vi "RP100 CLI Build.vi"(8 "Package Source Folder":path, 9 "Package Version":string="1.5.0.3") -> (0 "error out":errorcluster)   [LabVIEW 2019]
uses:
  <userlib>/LevyLab/Build Support/Build/Typedefs/Build Spec Type--combo.ctl
  <userlib>/LevyLab/Build Support/Build/Build.lvlib
panel:
  in  "error in":errorcluster
  out "project path":string
  out "repository path":string
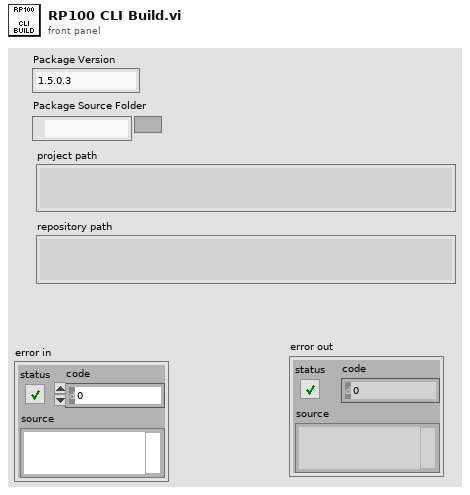
[diagram p1: front panel]
types:
  T1 = typedef "Build.lvlib/Build Spec Type--combo.ctl" = string
  T2 = typedef "Build.lvlib/Build Spec--cluster.ctl" = cluster{"Name":string, "Type":string, "Version":string}
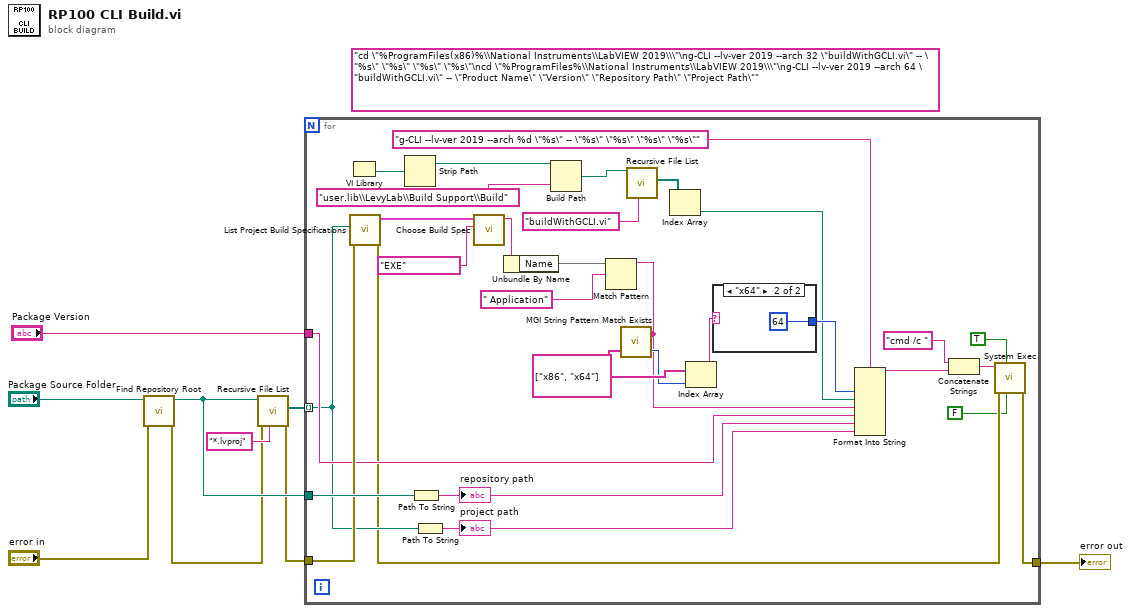
[diagram p0: block diagram]
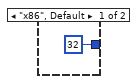
[diagram p2: hidden frame]
diagram:
  (unwired) "cd \"%ProgramFiles(x86)%\\National Instruments\\LabVIEW 2019\\\"\ng-CLI --lv-ver 2019 --arch 32 \"buildWithGCLI.vi\" -- \"%s\" \"%s\" \"%s\" \"%s\"\ncd \"%ProgramFiles%\\National Instruments\\LabVIEW 2019\\\"\ng-CLI --lv-ver 2019 --arch 64 \"buildWithGCLI.vi\" -- \"Product Name\" \"Version\" \"Repository Path\" \"Project Path\"" ("name or relative path")
  n1 = call "Find Repository Root.vi"("error in"="error in", "Package Source Folder"="Package Source Folder") -> ("error out"=w5:errorcluster, "repository path"=w6:path)  [unwired: 8 in]
  n2 = call <vilib>:"Recursive File List.vi"("pattern"="*.lvproj", "error in (no error)"=w5, "Folder Path"=w6) -> ("error out"=w4:errorcluster, "All Files in Dir"=w2:path[])  [unwired: 4 in, 3 out]
  n3 = for {
    tunnel: [w36] -> w9
    tunnel: w6 -> [w30]
    tunnel: w4 -> [w29]
    tunnel: "Package Version" -> [w28]
    tunnel: w2 -> [w27] mode=indexing
    w26 = string[] ["x86", "x64"] ("Patterns to Try")
    n4 = VI Library() -> (path=w13:path)
    n5 = call <userlib>:"List Project Build Specifications.vi"("error in (no error)"=w29, "project path"=w27) -> ("error out"=w22:errorcluster, "Build Specs"=w34:T2[])  [unwired: 8 in]
    n6 = Strip Path(path=w13) -> (stripped path=w12:path)  [unwired: 1 out]
    n7 = Path To String(path=w30) -> (string=w31:string)
    "repository path" <- w31
    n8 = Path To String(path=w27) -> (string=w32:string)
    "project path" <- w32
    n9 = call <userlib>:"Choose Build Spec.vi"("Build Type"=T1 "EXE", "Build Specs"=w34) -> ("Name"=w33:string)  [unwired: 6 in, 3 out]
    n10 = Unbundle By Name(w33) -> ("Name"=w20)
    n11 = Build Path(base path=w12, name or relative path="user.lib\\LevyLab\\Build Support\\Build") -> (appended path=w11:path)
    n12 = Match Pattern(string=w20, regular expression=" Application" ("format string")) -> (before substring=w19:string)  [unwired: 1 in, 3 out]
    n13 = call <userlib>:"MGI String Pattern Match Exists.vi"("Patterns to Try"=w26, "String"=w19) -> ("Index of First Pattern Matched"=w25:i32)  [unwired: 1 out]
    n14 = call <vilib>:"Recursive File List.vi"("pattern"="buildWithGCLI.vi", "Folder Path"=w11) -> ("All Files in Dir"=w14:path[])  [unwired: 5 in, 4 out]
    n15 = Index Array(array=w14) -> (element=w15:path)  [unwired: 1 in]
    n16 = Index Array(array=w26, index=w25) -> (element=w24:string)
    n17 = case shown="\"x64\"" w24 {
      tunnel: [32 64] -> w39
      frame "x86", Default {
      }
      frame "x64" {
      }
    }
    n18 = Format Into String(format string="g-CLI --lv-ver 2019 --arch %d \"%s\" -- \"%s\" \"%s\" \"%s\" \"%s\"" ("name or relative path"), w39, w15, w19, w28, w31, w32) -> (resulting string=w37:string)  [unwired: 2 in, 1 out]
    n19 = Concatenate Strings("cmd /c " ("name or relative path"), w37) -> (w23:string)
    n20 = call <vilib>:"System Exec.vi"("run minimized? (F)"=FALSE, "wait until completion? (T)"=TRUE, "error in (no error)"=w22, "command line"=w23) -> ("error out"=w36:errorcluster)  [unwired: 4 in, 3 out]
  }
  "error out" <- w9
